vi "4.5.vi"() -> ()   [LabVIEW 2017]
panel:
  out "循环次数":i32
  in  "指定值":dbl
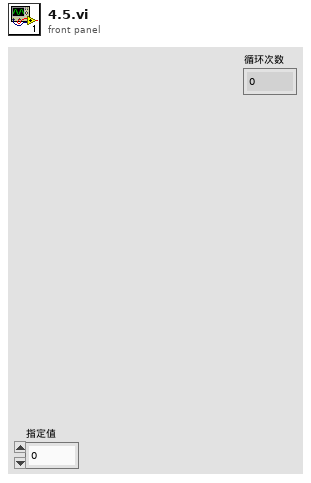
[diagram p1: front panel]
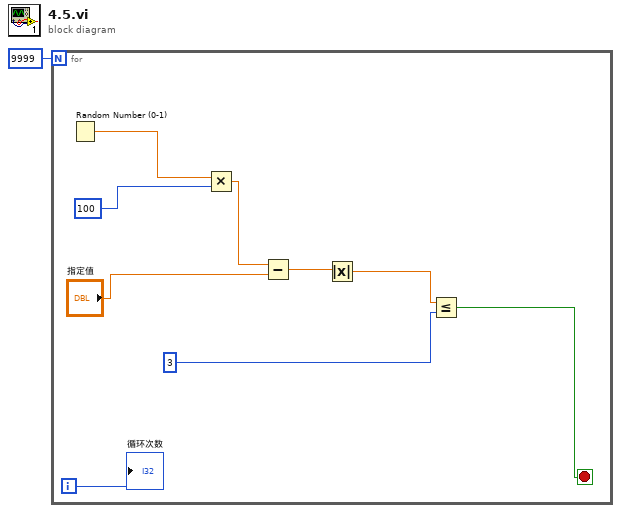
[diagram p0: block diagram]
diagram:
  n1 = for {
    N: 9999 -> [_]
    i -> [w8]
    stop <- w4 stop-if-true
    n2 = Random Number (0-1)() -> (number: 0 to 1=w10:dbl)
    n3 = Multiply(x=w10, y=100) -> (x*y=w6:dbl)
    n4 = Subtract(x=w6, y="指定值") -> (x-y=w5:dbl)
    n5 = Absolute Value(x=w5) -> (abs(x)=w3:dbl)
    n6 = Less Or Equal?(x=w3, y=3) -> (x <= y?=w4:bool)
    "循环次数" <- w8
  }
